vi "Initialize.vi"(8 "error in (no error)":errorcluster, 11 "IKA EUROSTAR Settings":T1) -> (0 "error out":errorcluster, 1 "Initialized":bool, 2 "Connection Error":bool, 3 "IKA EUROSTAR Settings":T1)   [LabVIEW 2021, in "IKA EUROSTAR.lvlib"]
uses:
  IKA EUROSTAR.lvlib
  IKA EUROSTAR Settings.ctl
  <vilib>/Instr/_visa.llb/VISA Configure Serial Port (Instr).vi
  support/Support Library.lvlib
panel:
  out "read buffer":string
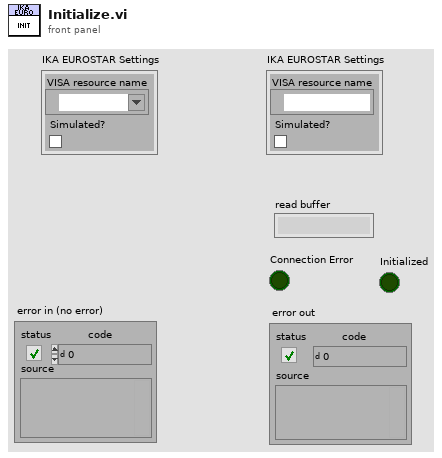
[diagram p1: front panel]
types:
  T1 = typedef "IKA EUROSTAR.lvlib/IKA EUROSTAR Settings.ctl" = cluster{"VISA resource name":refnum<visa-resource-name>, "Simulated?":bool}
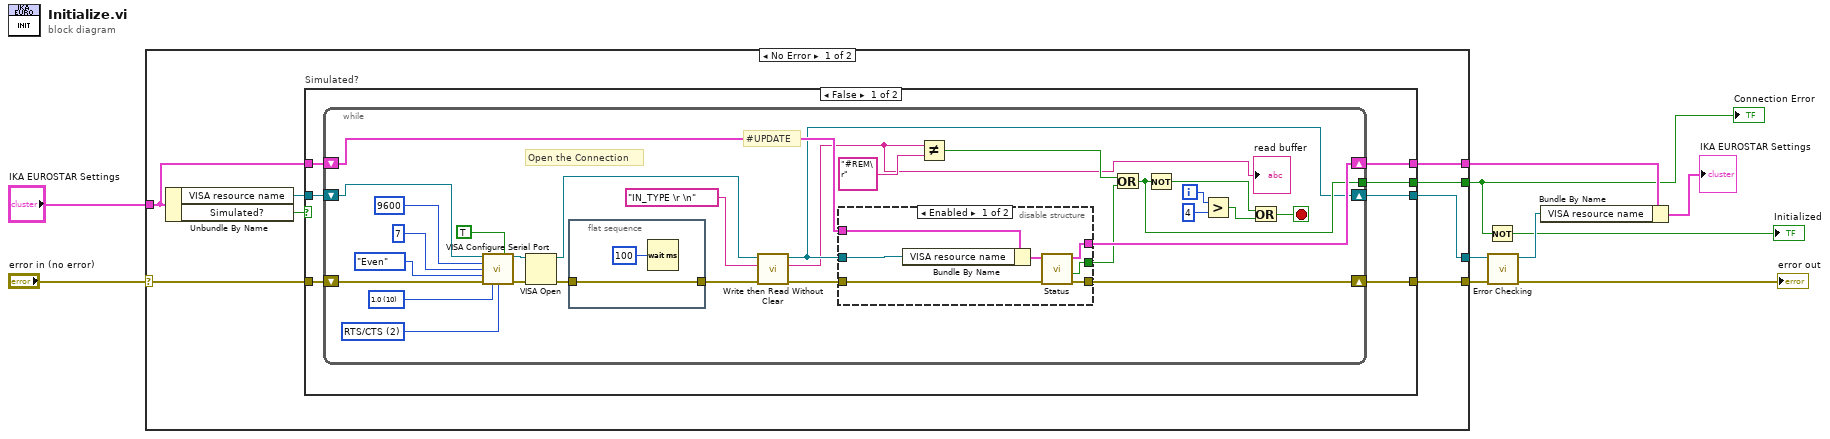
[diagram p0: block diagram]
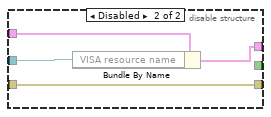
[diagram p2: hidden frame]
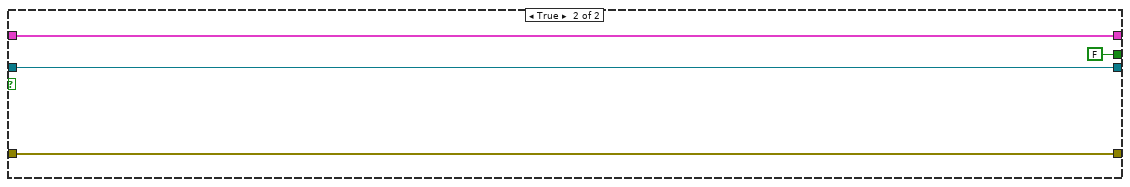
[diagram p3: hidden frame]
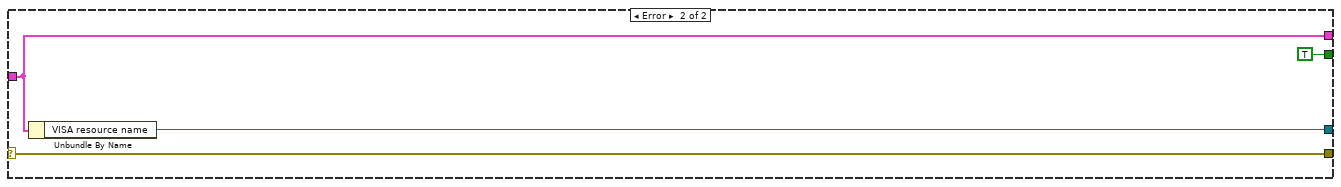
[diagram p4: hidden frame]
diagram:
  n1 = case shown="No Error" "error in (no error)" {
    selector: "error in (no error)" -> [w18 w75]
    tunnel: "IKA EUROSTAR Settings" -> [w12 w72]
    tunnel: [w17 w75] -> w8
    tunnel: [w15 w74] -> w9
    tunnel: [w13 TRUE] -> w3
    tunnel: [w11 w72] -> w5
    frame No Error {
      n2 = Unbundle By Name(w12) -> ("VISA resource name"=w16:refnum<visa-resource-name>, "Simulated?"=w14:bool)
      n3 = case "Simulated?" shown="False" w14 {
        tunnel: w18 -> [w25 w71]
        tunnel: [w21 w71] -> w17
        tunnel: [w19 w70] -> w15
        tunnel: w16 -> [w24 w70]
        tunnel: [w20 FALSE] -> w13
        tunnel: w12 -> [w23 w68]
        tunnel: [w22 w68] -> w11
        frame False {
          n4 = while {
            tunnel: [w37] -> w20
            shift-right: [w42] -> w21
            shift-left: w25 -> [w48]
            shift-right: [w28] -> w19
            shift-left: w24 -> [w46]
            shift-right: [w43] -> w22
            shift-left: w23 -> [w44]
            i -> [w34]
            stop <- w35 stop-if-true
            w50 = u16 2 items=["None", "XON/XOFF", "RTS/CTS", "XON/XOFF & RTS/CTS", "DTR/DSR", "XON/XOFF & DTR/DSR"] ("flow control (0:none)")
            w51 = u16 10 items=["1.0"=10, "1.5"=15, "2.0"=20] ("stop bits (10: 1 bit)")
            # "#UPDATE"
            # "Open the Connection"
            n5 = call-poly "VISA Configure Serial Port"("VISA resource name"=w46, "Enable Termination\nChar (T)"=TRUE ("Enable Termination\nChar (T)"), "baud rate (9600)"=u32 9600, "data bits (8)"=u16 7, "parity (0:none)"=enum16{"None", "Odd", "Even", "Mark", "Space"}."Even", "error in (no error)"=w48, "stop bits (10: 1 bit)"=w51, "flow control (0:none)"=w50) -> ("VISA resource name out"=w47:refnum<visa-resource-name>, "error out"=w49:errorcluster)  [unwired: 6 in]
            n6 = VISA Open(error in (no error)=w49, VISA resource name=w47) -> (VISA resource name=w31:refnum<visa-resource-name>, error out=w38:errorcluster)  [unwired: 3 in]
            n7 = flat-sequence {
              tunnel: [w67] -> w29
              tunnel: w38 -> [w67]
              frame #0 {
                n8 = Wait (ms)(milliseconds to wait=u32 100) -> ()  [unwired: 1 out]
              }
            }
            n9 = call "Write then Read Without Clear.vi"("error in"=w29, "write buffer"="IN_TYPE \r \n", "VISA resource name in"=w31) -> ("error out"=w26:errorcluster, "read buffer"=w27:string, "VISA resource name out"=w28:refnum<visa-resource-name>)  [unwired: 5 in, 1 out]
            "read buffer" <- w27
            n10 = disable-structure shown="Enabled" {
              disable-tunnel: w44 -> [w61 w64]
              disable-tunnel: [w59 w63] -> w43
              disable-tunnel: [w58 w65] -> w42
              disable-tunnel: [w57 _] -> w40
              disable-tunnel: w28 -> [w56 w62]
              disable-tunnel: w26 -> [w55 w65]
              frame Enabled {
                n11 = Bundle By Name(cluster=w61, "VISA resource name"=w56) -> (w60:T1)
                n12 = call "Status.vi"("error in (no error)"=w55, "IKA EUROSTAR Settings in"=w60) -> ("error out"=w58:errorcluster, "Connection Error"=w57:bool, "IKA EUROSTAR Settings Out"=w59:T1)  [unwired: 4 in, 3 out]
              }
              frame Disabled {
                n13 = Bundle By Name(cluster=w64, "VISA resource name"=w62) -> (w63:T1)
              }
            }
            n14 = Not Equal?(x=w27, y="#REM\r") -> (x != y?=w39:bool)
            n15 = Or(x=w39, y=w40) -> (x .or. y?=w37:bool)
            n16 = Not(x=w37) -> (.not. x?=w36:bool)
            n17 = Greater?(x=w34, y=4) -> (0:w32:bool)
            n18 = Or(x=w36, y=w32) -> (x .or. y?=w35:bool)
          }
        }
        frame True {
        }
      }
    }
    frame Error {
      n19 = Unbundle By Name(w72) -> ("VISA resource name"=w74:refnum<visa-resource-name>)
    }
  }
  "Connection Error" <- w3
  n20 = Not(x=w3) -> (.not. x?=→"Initialized":bool)
  n21 = call "Error Checking.vi"("error in (no error)"=w8, "VISA resource name"=w9) -> ("error out"=→"error out":errorcluster, "VISA resource name"=w6:refnum<visa-resource-name>)  [unwired: 7 in, 1 out]
  n22 = Bundle By Name(cluster=w5, "VISA resource name"=w6) -> (→"IKA EUROSTAR Settings":T1)
